vi "DAQmx Create Channel (CI-Count Edges).vi"(0 "task in":refnum<k21>, 1 "initial count":u32, 2 "count direction":i32(ring)=10128 items=["Count Up"=10128, "Count Down"=10124, "Externally Controlled"=10326], 3 "edge":i32(ring)=10280 items=["Rising"=10280, "Falling"=10171], 5 "counter":tag, 7 "name to assign":string, 11 "error in":errorcluster) -> (4 "task out":refnum<k21>, 15 "error out":errorcluster)   [LabVIEW 2013]
doc: "Creates a channel to count the number of rising or falling edges of a digital signal. You can create only one counter input channel at a time with this VI because a task can contain only one counter input channel. To read from multiple counters simultaneously, use a separate task for each counter. Connect the input signal to the default input terminal of the counter unless you select a different input terminal."
uses:
  C:/Program Files/National Instruments/LabVIEW 2013/resource/objmgr/daqmx.rc
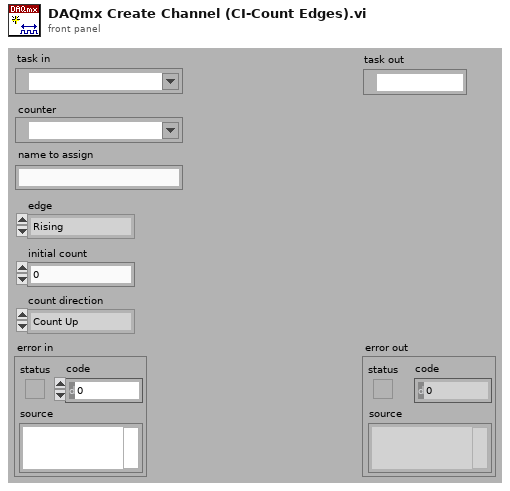
[diagram p1: front panel]
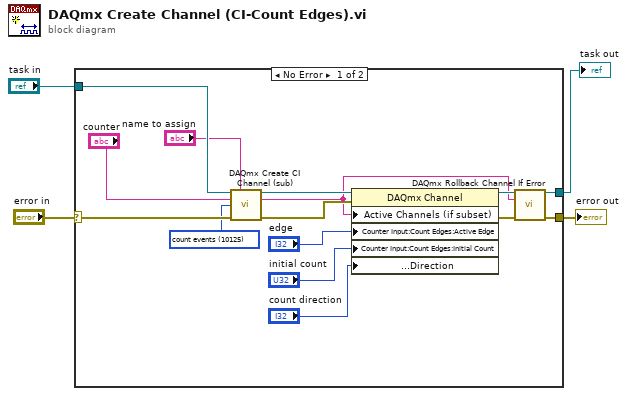
[diagram p0: block diagram]
diagram:
  n1 = case shown="No Error" "error in" {
    selector: "error in" -> [w18 w21]
    tunnel: [w7 w21] -> w4
    tunnel: "task in" -> [w19 w20]
    tunnel: [w8 w20] -> w1
    frame No Error {
      w12 = 10125 items=["count events"=10125, "frequency"=10179, "period"=10256, "pulse width"=10267, "semi period"=10289] ("measurement type")
      n2 = call "DAQmx Create CI Channel (sub).vi"("task in"=w19, "virtual channel name"="name to assign", "physical channel name"="counter", "measurement type"=w12, "error in"=w18) -> ("task out"=w10:refnum<k21>, "channel names"=w5:string, "error out"=w16:errorcluster)  [unwired: 1 in, 7 out]
      n3 = property class="DAQmx Channel"(reference=w10, error in=w16, "Active Channels (if subset)"=w5, "Counter Input:Count Edges:Active Edge"="edge", "Counter Input:Count Edges:Initial Count"="initial count", "Counter Input:Count Edges:Count Direction:Direction"="count direction") -> (reference out=w9:refnum<k21>, error out=w6:errorcluster)
      n4 = call "DAQmx Rollback Channel If Error.vi"("task in"=w9, "channel names"=w5, "error in"=w6) -> ("task out"=w8:refnum<k21>, "error out"=w7:errorcluster)  [unwired: 11 out]
    }
    frame Error {
    }
  }
  "error out" <- w4
  "task out" <- w1
